vi "Custom Assertion Failure Message.vi"() -> ()   [LabVIEW 2017, in "Assertions.Tests.lvlib" / "Assert Error Message Contains String.lvlib"]
uses:
  Assert Error Message Contains String.lvlib
  217b4f57-2f31-42df-b5ae-10c04b4f12b7.vi
  src/Transparent Assertions/Constraints/IsEqual/Create.vi
  src/Transparent Assertions/Constraints/IsEqual/IsEqual.lvclass
  src/Transparent Assertions/Assertions/Assertions.lvlib
  Assertions.Tests.lvlib
panel:
  out "error out":errorcluster
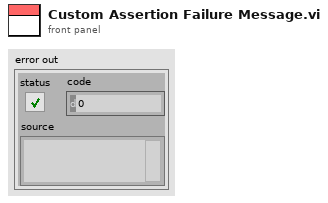
[diagram p1: front panel]
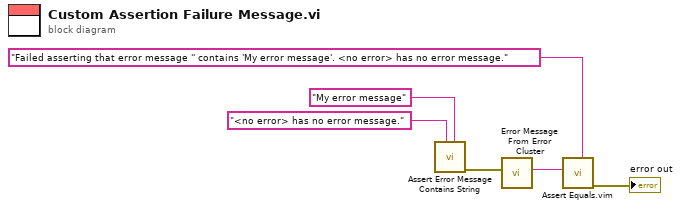
[diagram p0: block diagram]
diagram:
  n1 = call "Assert Error Message Contains String.vi"("Expected"="My error message", "Message (\"\")"="<no error> has no error message." ("Message (\"\")")) -> ("error out"=w2:errorcluster)  [unwired: 9 in]
  n2 = call "Error Message From Error Cluster.vi"("Error"=w2) -> ("Error Message"=w1:string)  [unwired: 10 in]
  n3 = call "Assert Equals.vim"("Expected"="Failed asserting that error message '' contains 'My error message'. <no error> has no error message." ("Needle"), "Actual"=w1) -> ("error out"=→"error out":errorcluster)  [unwired: 9 in]
